vi "limit phase to 180 degrees.vi"(8 "enable":bool, 10 "phase in":dbl, 11 "gain in":dbl) -> (2 "phase out":dbl, 3 "gain out":dbl)   [LabVIEW 2016]
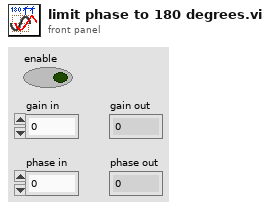
[diagram p1: front panel]
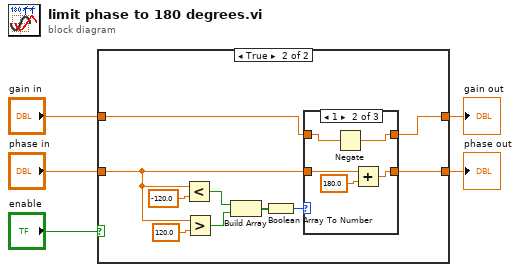
[diagram p0: block diagram]
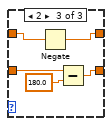
[diagram p4: hidden frame]
diagram:
  n1 = case shown="True" "enable" {
    tunnel: [w7 w17] -> w5
    tunnel: "gain in" -> [w7 w16]
    tunnel: [w6 w15] -> w3
    tunnel: "phase in" -> [w6 w14]
    frame False {
    }
    frame True {
      n2 = Less?(x=w14, y=-120.0) -> (x < y?=w11:bool)
      n3 = Greater?(x=w14, y=120.0) -> (0:w10:bool)
      n4 = Build Array(w11, w10) -> (w12:bool[])
      n5 = Boolean Array To Number(Boolean array=w12) -> (number=w13:u32)
      n6 = case shown="1" w13 {
        tunnel: w14 -> [w19 w24 w29]
        tunnel: [w19 w22 w27] -> w15
        tunnel: w16 -> [w18 w21 w26]
        tunnel: [w18 w20 w25] -> w17
        frame 0, Default {
        }
        frame 1 {
          n7 = Negate(x=w21) -> (-x=w20:dbl)
          n8 = Add(x=w24, y=180.0) -> (x+y=w22:dbl)
        }
        frame 2 {
          n9 = Negate(x=w26) -> (-x=w25:dbl)
          n10 = Subtract(x=w29, y=180.0) -> (x-y=w27:dbl)
        }
      }
    }
  }
  "gain out" <- w5
  "phase out" <- w3
